vi "Calculate Left Movement.vi"(8 "Camera Speed":sgl, 9 "Rotation":sgl, 10 "Previous Left":sgl, 11 "Previous Forward":sgl) -> (2 "Next Left":sgl, 3 "Next Forward":sgl)   [LabVIEW 2020, in "Scene.lvclass"]
uses:
  Scene.lvclass
  Scene.lvclass/Scene.ctl
  Graphics/Libraries/3D/3D.lvlib
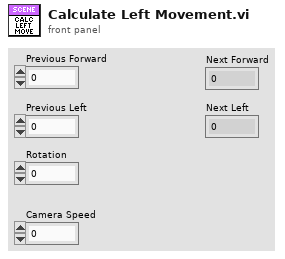
[diagram p1: front panel]
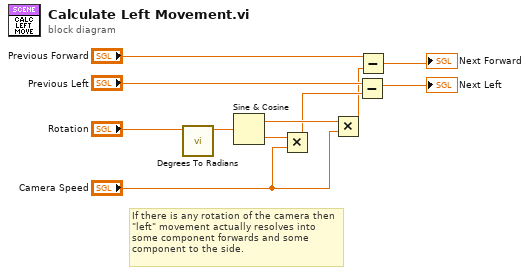
[diagram p0: block diagram]
diagram:
  # "If there is any rotation of the camera then \"left\" movement actually resolves into some component forwards and some component to the side."
  n1 = call "Degrees To Radians.vi"("Angle (°)"="Rotation") -> ("Angle (rad)"=w8:sgl)  [unwired: 10 in]
  n2 = Sine & Cosine(0:w8) -> (1:w7:sgl, 2:w5:sgl)
  n3 = Multiply(x=w5, y="Camera Speed") -> (x*y=w3:sgl)
  n4 = Multiply(x=w7, y="Camera Speed") -> (x*y=w2:sgl)
  n5 = Subtract(x="Previous Left", y=w3) -> (x-y=→"Next Left":sgl)
  n6 = Subtract(x="Previous Forward", y=w2) -> (x-y=→"Next Forward":sgl)
